vi "Update Step Parameters.vi"(8 "error in":errorcluster, 9 "Old Values":T1, 10 "New Values":T1, 11 "Plugin in":refnum<class "Sequencer with Output Values.lvclass">) -> (0 "error out":errorcluster, 2 "Step Values":T2[](array[typedef]), 3 "Plugin out":refnum<class "Sequencer with Output Values.lvclass">)   [LabVIEW 2024, in "Sequencer with Output Values.lvlib" / "Sequencer with Output Values.lvclass"]
uses:
  Sequencer with Output Values.lvclass
  C:/Program Files/National Instruments/LabVIEW 2024/vi.lib/FlexLogger/SDK/PluginSDK.lvlibp/PEFClasses/SDK/Plugin/Plugin.lvclass
  Step Settings.ctl
  Global Strings.vi
  <vilib>/FlexLogger/SDK/PluginSDK.lvlibp/PEFClasses/SDK/Plugin/ParameterAccess/Read DBL.vi
  <vilib>/FlexLogger/SDK/PluginSDK.lvlibp/PEFClasses/SDK/Plugin/ParameterAccess/Read Enum.vi
  <vilib>/FlexLogger/SDK/PluginSDK.lvlibp/PEFClasses/SDK/Plugin/ParameterAccess/Write Enum.vi
  <vilib>/FlexLogger/SDK/PluginSDK.lvlibp/PEFClasses/SDK/Plugin/ParameterAccess/Write DBL.vi
  <vilib>/FlexLogger/SDK/PluginSDK.lvlibp/PEFClasses/SDK/Plugin/Plugin.lvclass
  C:/Program Files/National Instruments/LabVIEW 2024/vi.lib/FlexLogger/SDK/PluginSDK.lvlibp/PEFClasses/SDK/Processing Element/Processing Element.lvclass
  C:/dev/niflexlogger-plugins/plugins/Sequencer with Output Values/source/Sequencer with Output Values/Sequencer with Output Values.lvclass
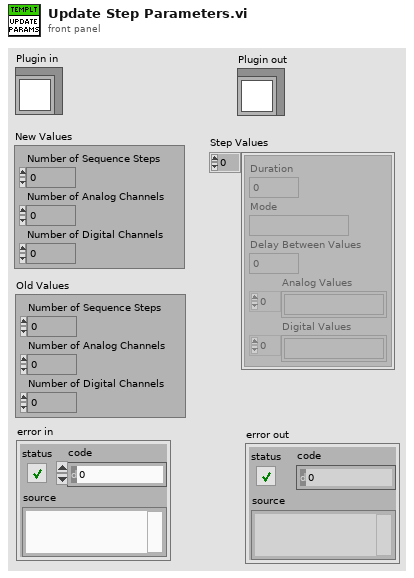
[diagram p1: front panel]
types:
  T1 = cluster{"Number of Sequence Steps":i32, "Number of Analog Channels":i32, "Number of Digital Channels":i32}
  T2 = typedef "Step Settings.ctl" = cluster{"Duration":dbl, "Mode":string, "Delay Between Values":dbl, "Analog Values":string[], "Digital Values":string[]}
  T3 = cluster{"f":dbl, "Value":string, "Value":dbl, "Values":string[], "Values":string[]}
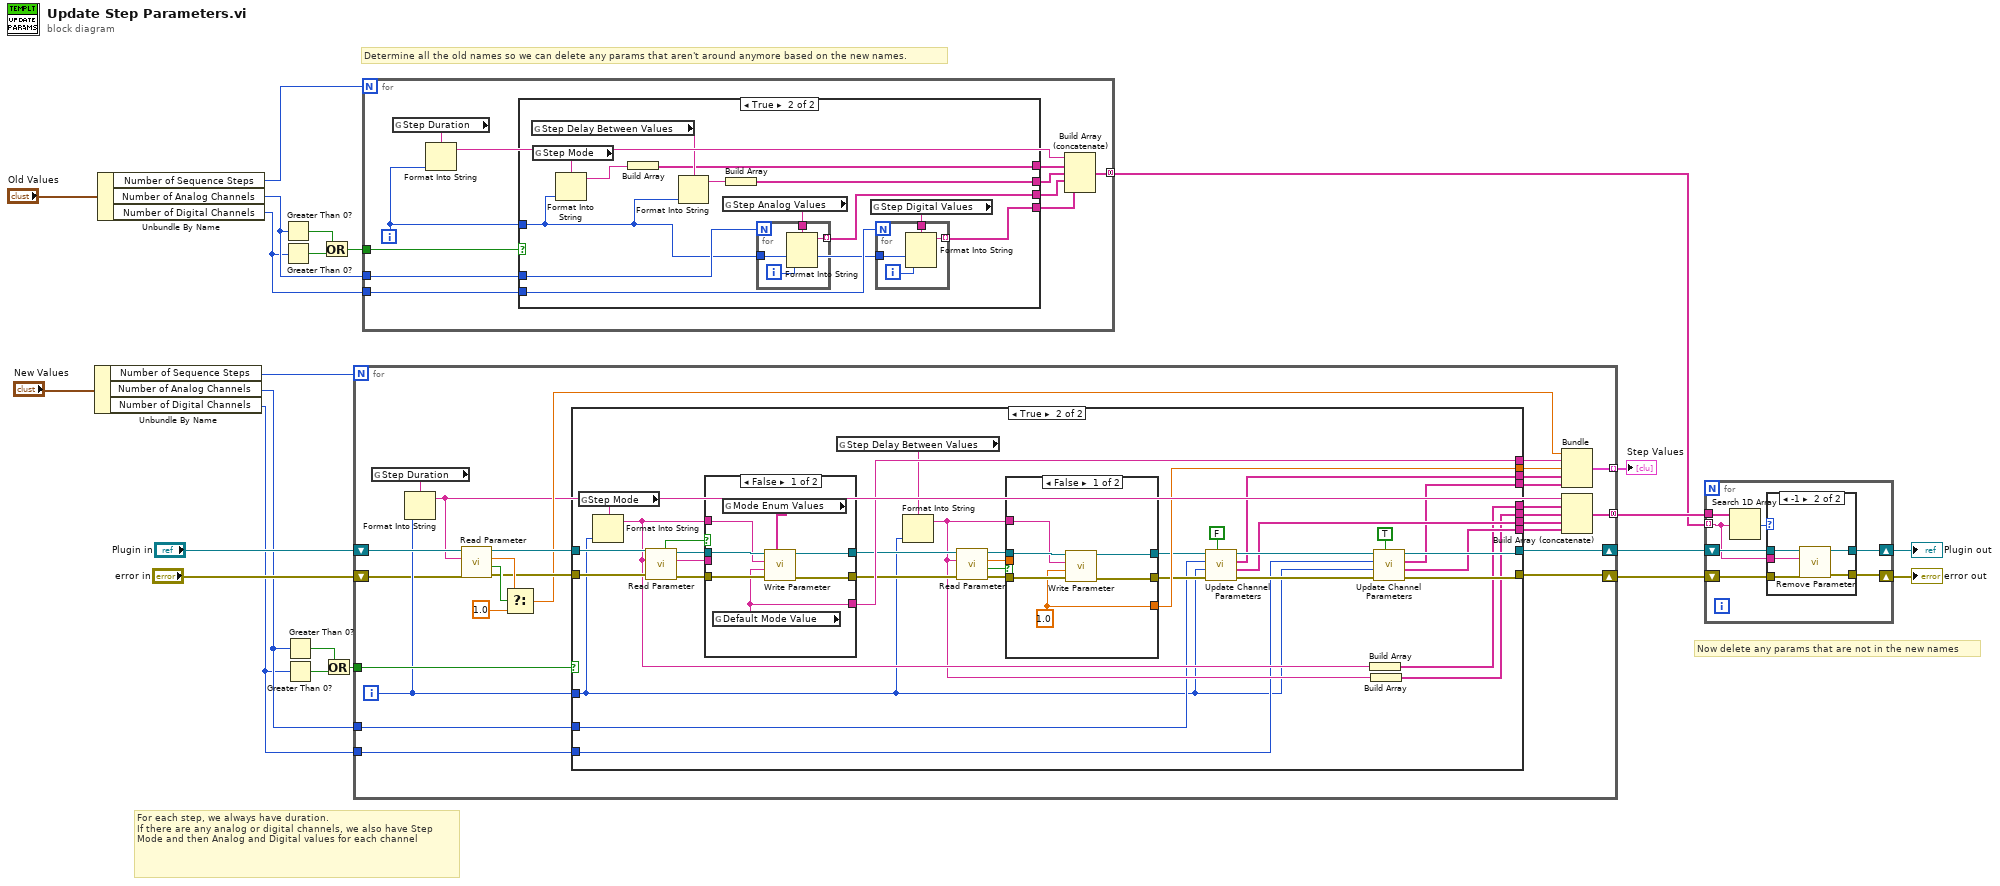
[diagram p0: block diagram]
diagram:
  # "Now delete any params that are not in the new names"
  # "Determine all the old names so we can delete any params that aren't around anymore based on the new names."
  # "For each step, we always have duration.\nIf there are any analog or digital channels, we also have Step Mode and then Analog and Digital values for each channel"
  n1 = Unbundle By Name("New Values") -> ("Number of Sequence Steps"=w16:i32, "Number of Analog Channels"=w15:i32, "Number of Digital Channels"=w14:i32)
  n2 = Unbundle By Name("Old Values") -> ("Number of Sequence Steps"=w12:i32, "Number of Analog Channels"=w8:i32, "Number of Digital Channels"=w7:i32)
  n3 = Greater Than 0?(x=w8) -> (x > 0?=w11:bool)
  n4 = Greater Than 0?(x=w7) -> (x > 0?=w10:bool)
  n5 = Greater Than 0?(x=w15) -> (x > 0?=w23:bool)
  n6 = Greater Than 0?(x=w14) -> (x > 0?=w22:bool)
  n7 = Or(x=w11, y=w10) -> (x .or. y?=w9:bool)
  n8 = Or(x=w23, y=w22) -> (x .or. y?=w21:bool)
  n9 = for {
    N: w16 -> [_]
    tunnel: w21 -> [w43]
    shift-right: [w40] -> w6
    shift-left: "Plugin in" -> [w45]
    tunnel: w14 -> [w36]
    tunnel: w15 -> [w35]
    tunnel: [w27] -> w18 mode=indexing
    tunnel: [w26] -> w4 mode=concatenating
    shift-right: [w25] -> w5
    shift-left: "error in" -> [w24]
    i -> [w41]
    n10 = global read "Global Strings.vi" "Step Duration"() -> (w46:string)
    n11 = Format Into String(format string=w46, w41) -> (resulting string=w34:string)  [unwired: 2 in, 1 out]
    n12 = call-poly <vilib>:"Read Parameter.vi"("error in (no error)"=w24, "Name"=w34, "Plugin in"=w45) -> ("error out"=w42:errorcluster, "Found"=w49:bool, "Value"=w48:dbl, "Plugin out"=w44:refnum<class "Sequencer with Output Values.lvclass">)  [unwired: 5 in]
    n13 = Select(t=w48, s=w49, f=1.0) -> (s? t:f=w39:dbl)
    n14 = case shown="True" w43 {
      tunnel: w44 -> [w51 w86]
      tunnel: w42 -> [w50 w82]
      tunnel: w41 -> [_ w62]
      tunnel: [w51 w61] -> w40
      tunnel: [w50 w60] -> w25
      tunnel: [_ w80] -> w38
      tunnel: [_ w71] -> w37
      tunnel: w36 -> [_ w63]
      tunnel: w35 -> [_ w64]
      tunnel: [_ w55] -> w33
      tunnel: [_ w54] -> w32
      tunnel: [_ w59] -> w31
      tunnel: [_ w58] -> w30
      tunnel: [_ w57] -> w29
      tunnel: [_ w56] -> w28
      frame False {
      }
      frame True {
        n15 = global read "Global Strings.vi" "Step Mode"() -> (w74:string)
        n16 = Format Into String(format string=w74, w62) -> (resulting string=w68:string)  [unwired: 2 in, 1 out]
        n17 = call-poly <vilib>:"Read Parameter.vi"("error in (no error)"=w82, "Name"=w68, "Plugin in"=w86) -> ("error out"=w81:errorcluster, "Value"=w83:string, "Plugin out"=w84:refnum<class "Sequencer with Output Values.lvclass">, "Found"=w85:bool)  [unwired: 4 in, 1 out]
        n18 = case shown="False" w85 {
          tunnel: w84 -> [w102 w104]
          tunnel: w68 -> [w101 _]
          tunnel: w83 -> [_ w105]
          tunnel: w81 -> [w100 w103]
          tunnel: [w98 w105] -> w80
          tunnel: [w97 w104] -> w79
          tunnel: [w96 w103] -> w78
          frame False {
            n19 = global read "Global Strings.vi" "Default Mode Value"() -> (w98:string)
            n20 = global read "Global Strings.vi" "Mode Enum Values"() -> (w99:string[])
            n21 = call-poly <vilib>:"Write Parameter.vi"("Possible Values"=w99, "error in (no error)"=w100, "Current Value"=w98, "Name"=w101, "Plugin in"=w102) -> ("error out"=w96:errorcluster, "Plugin out"=w97:refnum<class "Sequencer with Output Values.lvclass">)  [unwired: 5 in]
          }
          frame True {
          }
        }
        n22 = global read "Global Strings.vi" "Step Delay Between Values"() -> (w73:string)
        n23 = Format Into String(format string=w73, w62) -> (resulting string=w67:string)  [unwired: 2 in, 1 out]
        n24 = call-poly <vilib>:"Read Parameter.vi"("error in (no error)"=w78, "Name"=w67, "Plugin in"=w79) -> ("error out"=w76:errorcluster, "Found"=w75:bool, "Value"=w72:dbl, "Plugin out"=w77:refnum<class "Sequencer with Output Values.lvclass">)  [unwired: 5 in]
        n25 = case shown="False" w75 {
          tunnel: w77 -> [w92 w95]
          tunnel: w76 -> [w91 w94]
          tunnel: [w90 w95] -> w70
          tunnel: [w89 w94] -> w69
          tunnel: w67 -> [w88 _]
          tunnel: w72 -> [_ w93]
          tunnel: [w87 w93] -> w71
          frame False {
            w87 = 1.0 ("Value")
            n26 = call-poly <vilib>:"Write Parameter.vi"("error in (no error)"=w91, "Value"=w87, "Name"=w88, "Plugin in"=w92) -> ("error out"=w89:errorcluster, "Plugin out"=w90:refnum<class "Sequencer with Output Values.lvclass">)  [unwired: 6 in]
          }
          frame True {
          }
        }
        n27 = call "Update Channel Parameters.vi"("Digital"=FALSE, "error in (no error)"=w69, "Sequence Number"=w62, "Number of Channels"=w64, "Plugin in"=w70) -> ("error out"=w65:errorcluster, "Names"=w58:string[], "Values"=w57:string[], "Plugin out"=w66:refnum<class "Sequencer with Output Values.lvclass">)  [unwired: 3 in]
        n28 = Build Array(w68) -> (w55:string[])
        n29 = Build Array(w67) -> (w54:string[])
        n30 = call "Update Channel Parameters.vi"("Digital"=TRUE, "error in (no error)"=w65, "Sequence Number"=w62, "Number of Channels"=w63, "Plugin in"=w66) -> ("error out"=w60:errorcluster, "Names"=w59:string[], "Values"=w56:string[], "Plugin out"=w61:refnum<class "Sequencer with Output Values.lvclass">)  [unwired: 3 in]
      }
    }
    n31 = Bundle("f"=w39, "Value"=w38, "Value"=w37, "Values"=w29, "Values"=w28) -> (w27:T3)  [unwired: 1 in]
    n32 = Build Array (concatenate)(w34, w33, w32, w30, w31) -> (w26:string[])
  }
  "Step Values" <- w18
  n33 = for {
    N: w12 -> [_]
    tunnel: w9 -> [w115]
    tunnel: w8 -> [w113]
    tunnel: w7 -> [w112]
    tunnel: [w106] -> w3 mode=concatenating
    i -> [w114]
    n34 = global read "Global Strings.vi" "Step Duration"() -> (w116:string)
    n35 = Format Into String(format string=w116, w114) -> (resulting string=w110:string)  [unwired: 2 in, 1 out]
    n36 = case shown="True" w115 {
      tunnel: w114 -> [_ w119]
      tunnel: [_ w126] -> w111
      tunnel: w113 -> [_ w123]
      tunnel: [_ w124] -> w109
      tunnel: [_ w121] -> w108
      tunnel: w112 -> [_ w120]
      tunnel: [_ w117] -> w107
      frame False {
      }
      frame True {
        n37 = global read "Global Strings.vi" "Step Delay Between Values"() -> (w127:string)
        n38 = global read "Global Strings.vi" "Step Mode"() -> (w129:string)
        n39 = Format Into String(format string=w129, w119) -> (resulting string=w128:string)  [unwired: 2 in, 1 out]
        n40 = Build Array(w128) -> (w126:string[])
        n41 = Format Into String(format string=w127, w119) -> (resulting string=w125:string)  [unwired: 2 in, 1 out]
        n42 = global read "Global Strings.vi" "Step Analog Values"() -> (w122:string)
        n43 = Build Array(w125) -> (w124:string[])
        n44 = for {
          N: w123 -> [_]
          tunnel: w119 -> [w136]
          tunnel: w122 -> [w135]
          tunnel: [w134] -> w121 mode=indexing
          i -> [w137]
          n45 = Format Into String(format string=w135, w136, w137) -> (resulting string=w134:string)  [unwired: 2 in, 1 out]
        }
        n46 = global read "Global Strings.vi" "Step Digital Values"() -> (w118:string)
        n47 = for {
          N: w120 -> [_]
          tunnel: w119 -> [w132]
          tunnel: w118 -> [w131]
          tunnel: [w130] -> w117 mode=indexing
          i -> [w133]
          n48 = Format Into String(format string=w131, w132, w133) -> (resulting string=w130:string)  [unwired: 2 in, 1 out]
        }
      }
    }
    n49 = Build Array (concatenate)(w110, w111, w109, w108, w107) -> (w106:string[])
  }
  n50 = for {
    tunnel: w4 -> [w144]
    tunnel: w3 -> [w141] mode=indexing
    shift-right: [w139] -> w2
    shift-left: w6 -> [w142]
    shift-right: [w138] -> w1
    shift-left: w5 -> [w140]
    n51 = Search 1D Array(1D array=w144, element=w141) -> (index of element=w143:i32)  [unwired: 1 in]
    n52 = case shown="-1" w143 {
      tunnel: w142 -> [w146 w151]
      tunnel: w141 -> [_ w150]
      tunnel: w140 -> [w145 w149]
      tunnel: [w146 w148] -> w139
      tunnel: [w145 w147] -> w138
      frame 0, Default {
      }
      frame -1 {
        n53 = call <vilib>:"Remove Parameter.vi"("error in (no error)"=w149, "Name"=w150, "Plugin in"=w151) -> ("error out"=w147:errorcluster, "Plugin out"=w148:refnum<class "Sequencer with Output Values.lvclass">)  [unwired: 7 in]
      }
    }
  }
  "Plugin out" <- w2
  "error out" <- w1
